vi "初始化移位寄存器.vi"() -> ()   [LabVIEW 2009]
panel:
  in  "循环次数i":i32
  out "i次循环后数据":i32
  out "第i-3次迭代数据":i32
  out "第i-2次迭代数据":i32
  out "第i-1次迭代数据":i32
  out "数值":i32
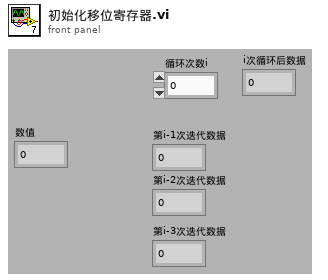
[diagram p1: front panel]
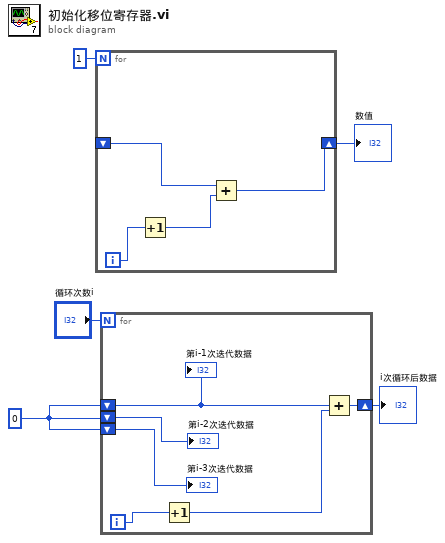
[diagram p0: block diagram]
diagram:
  w1 = 0
  n1 = for {
    N: 1 -> [_]
    shift-right: [w8] -> w4
    shift-left: _ -> [w9]
    i -> [w7]
    n2 = Increment(x=w7) -> (x+1=w6:i32)
    n3 = Add(x=w9, y=w6) -> (x+y=w8:i32)
  }
  "数值" <- w4
  n4 = for {
    N: "循环次数i" -> [_]
    shift-right: [w14] -> w3
    shift-left: w1 -> [w15]
    shift-left: w1 -> [w11]
    shift-left: w1 -> [w10]
    i -> [w13]
    n5 = Increment(x=w13) -> (x+1=w12:i32)
    n6 = Add(x=w15, y=w12) -> (x+y=w14:i32)
    "第i-1次迭代数据" <- w15
    "第i-2次迭代数据" <- w11
    "第i-3次迭代数据" <- w10
  }
  "i次循环后数据" <- w3
